vi "Write Configuration.vi"(7 "Section":string, 8 "error in (no error)":errorcluster, 10 "Offset":dbl[](array[numeric]), 11 "Product":string) -> (0 "error out":errorcluster)   [LabVIEW 2013]
uses:
  <vilib>/Utility/config.llb/Write Key (String).vi
  <vilib>/Utility/config.llb/Write Key (Double).vi
  <vilib>/Utility/config.llb/NI_LVConfig.lvlib
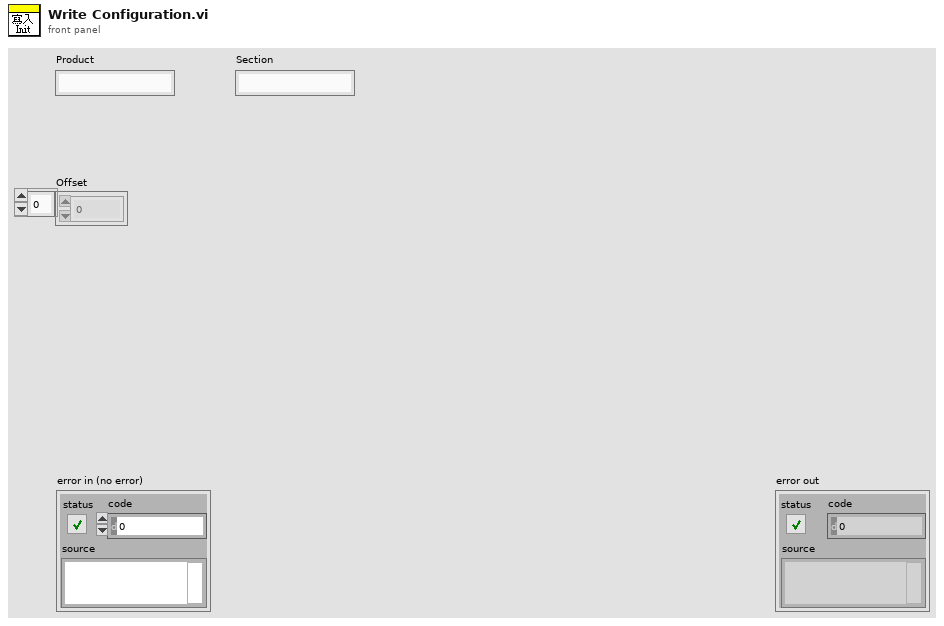
[diagram p1: front panel]
types:
  T1 = typedef "NI_LVConfig.lvlib/Config Data RefNum.ctl" = refnum<k1>
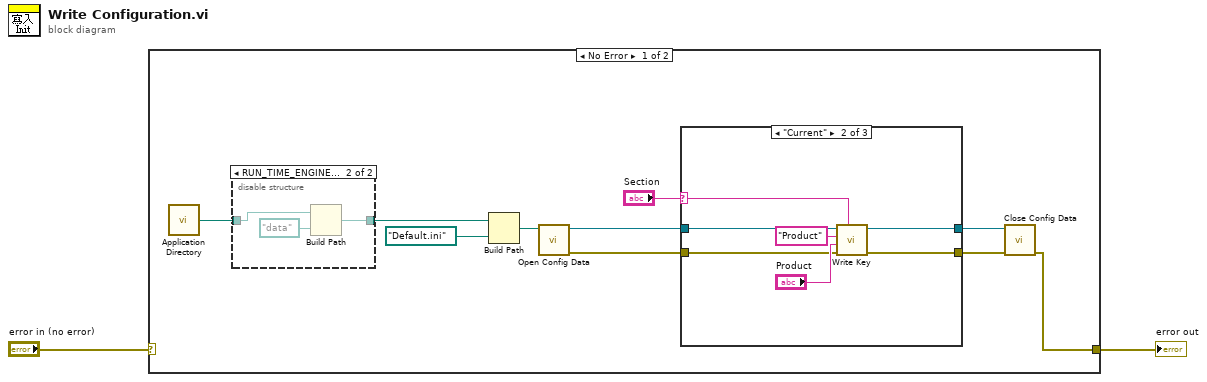
[diagram p0: block diagram]
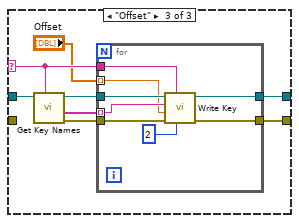
[diagram p3: hidden frame]
diagram:
  n1 = case shown="No Error" "error in (no error)" {
    selector: "error in (no error)" -> [_ w42]
    tunnel: [w8 w42] -> w1
    frame No Error {
      n2 = call <vilib>:"Application Directory.vi"() -> ("Application Directory"=w12:path)
      n3 = disable-structure shown="RUN_TIME_ENGINE==True" {
        disable-tunnel: [w38 w40] -> w11
        disable-tunnel: w12 -> [w38 w39]
        frame condition #0 (active) {
        }
        frame condition #1 {
          n4 = Build Path(base path=w39, name or relative path=path "data") -> (appended path=w40:path)
        }
      }
      n5 = Build Path(base path=w11, name or relative path=path "Default.ini") -> (appended path=w10:path)
      n6 = call <vilib>:"Open Config Data.vi"("configuration file path"=w10) -> ("error out"=w4:errorcluster, "refnum"=w7:T1)  [unwired: 8 in, 1 out]
      n7 = case shown="\"Current\"" "Section" {
        selector: "Section" -> [_ w21 w26]
        tunnel: w7 -> [w14 w18 w24]
        tunnel: [w14 w15 w23] -> w6
        tunnel: [w13 w16 w22] -> w5
        tunnel: w4 -> [w13 w17 _]
        frame Default {
        }
        frame "Current" {
          n8 = call-poly <vilib>:"Write Key.vi"("section"=w21, "error in (no error)"=w17, "value"="Product", "key"="Product", "refnum"=w18) -> ("error out"=w16:errorcluster, "refnum out"=w15:T1)  [unwired: 4 in, 1 out]
        }
        frame "Offset" {
          n9 = call <vilib>:"Get Key Names.vi"("section"=w26, "refnum"=w24) -> ("error out"=w27:errorcluster, "key names"=w29:string[], "refnum out"=w28:T1)  [unwired: 6 in, 1 out]
          n10 = for {
            tunnel: w29 -> [w34] mode=indexing
            tunnel: w26 -> [w37]
            tunnel: w28 -> [w36]
            tunnel: w27 -> [w35]
            tunnel: "Offset" -> [w33] mode=indexing
            tunnel: [w32] -> w23
            tunnel: [w31] -> w22
            n11 = call-poly <vilib>:"Write Key.vi"("precision (6)"=i16 2, "section"=w37, "error in (no error)"=w35, "value"=w33, "key"=w34, "refnum"=w36) -> ("error out"=w31:errorcluster, "refnum out"=w32:T1)  [unwired: 3 in, 1 out]
          }
        }
      }
      n12 = call <vilib>:"Close Config Data.vi"("error in (no error)"=w5, "refnum"=w6) -> ("error out"=w8:errorcluster)  [unwired: 8 in, 1 out]
    }
    frame Error {
    }
  }
  "error out" <- w1
